vi "Close.vi"(8 "error in (no error)":errorcluster, 11 "Arinst SSA-TG in":refnum<class "PL Arinst SSA-TG.lvclass">) -> (0 "error out":errorcluster)   [LabVIEW 2015, in "PL Arinst SSA-TG.lvclass"]
doc: "Closes connection to device."
uses:
  PL Arinst SSA-TG.lvclass
  PL Arinst SSA-TG.lvclass/PL Arinst SSA-TG.ctl
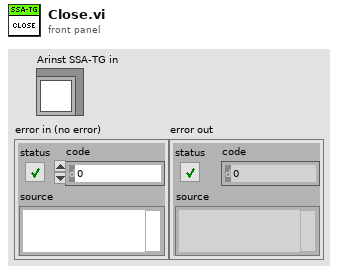
[diagram p1: front panel]
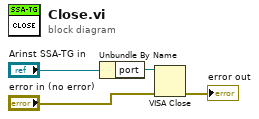
[diagram p0: block diagram]
diagram:
  n1 = Unbundle By Name("Arinst SSA-TG in") -> ("port"=w3:refnum<visa-resource-name>)
  n2 = VISA Close(VISA resource name=w3, error in (no error)="error in (no error)") -> (error out=→"error out":errorcluster)
